vi "Copy All.vi"(8 "error in (no error)":errorcluster, 10 "dst Pointer in":refnum<class "Pointer.lvclass">, 11 "src Pointer in":refnum<class "Pointer.lvclass">) -> (0 "error out":errorcluster, 2 "dst Pointer out":refnum<class "Pointer.lvclass">, 3 "src Pointer out":refnum<class "Pointer.lvclass">)   [LabVIEW 2017, in "Memory Manager.lvlib" / "Pointer.lvclass"]
doc: "Copies all of the data from the memory address specified by <b>src pointer</b> to the memory address specified by <b>dst pointer</b>.\n\n<b>Note:</b> This VI is <b>safe</b>.\n\nSafe means that this function evaluates that the size parameter of <b>dst pointer</b> is greater than or equal to the size of <b>src pointer</b> to ensure that the destination memory location is an appropriate size before copying data from source to destination. Reading/writing more data to a pointer than it has allocated can corrupt or crash LabVIEW."
uses:
  Pointer.lvclass
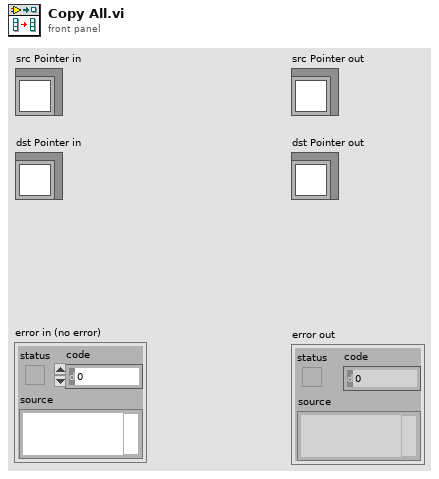
[diagram p1: front panel]
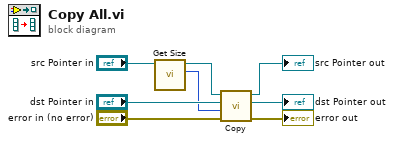
[diagram p0: block diagram]
diagram:
  n1 = call "Get Size.vi"("Pointer in"="src Pointer in") -> ("size"=w5:u64, "Pointer out"=w7:refnum<class "Pointer.lvclass">)  [unwired: 9 in]
  n2 = call "Copy.vi"("error in (no error)"="error in (no error)", "bytes to copy"=w5, "dst Pointer in"="dst Pointer in", "src Pointer in"=w7) -> ("error out"=→"error out":errorcluster, "dst Pointer out"=→"dst Pointer out":refnum<class "Pointer.lvclass">, "src Pointer out"=→"src Pointer out":refnum<class "Pointer.lvclass">)  [unwired: 4 in, 1 out]
